vi "Drive Begin.vi"() -> ()   [LabVIEW 2016]
uses:
  <vilib>/Rock Robotics/WPI/Joystick/WPI_JoystickDeviceEnum.ctl
  <vilib>/Rock Robotics/SystemInterfaces/DIO/FPGA_DIOChannel.ctl
  <vilib>/Rock Robotics/WPI/Encoder/WPI_EncoderType.ctl
  <vilib>/Rock Robotics/SystemInterfaces/DIO/FPGA_DIOPWMChannel.ctl
  <vilib>/Rock Robotics/WPI/SafetyOutput/WPI_SafetyOutputConfigMenu.ctl
  <vilib>/Rock Robotics/WPI/Counter/WPI_CounterDigitalInputToDigitalSource.vi
  <vilib>/Rock Robotics/WPI/Utilities/WPI_GetSetVariantRefNum.vi
  <vilib>/Rock Robotics/WPI/RobotDrive/WPI_RobotDriveOpen2MotorWithVictorSP.vi
  <vilib>/Rock Robotics/WPI/Solenoid/WPI_SolenoidChannel.ctl
  <vilib>/Rock Robotics/WPI/Solenoid/WPI_SolenoidOpenSingle.vi
panel:
  out "error out":errorcluster
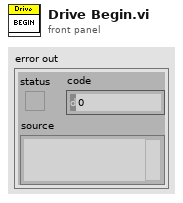
[diagram p1: front panel]
types:
  T1 = typedef "WPI_SafetyOutputConfigMenu.ctl" = enum16{"Enable", "Disable"}
  T2 = typedef "FPGA_DIOPWMChannel.ctl" = enum8{"PWM 0", "PWM 1", "PWM 2", "PWM 3", "PWM 4", "PWM 5", "PWM 6", "PWM 7", "PWM 8", "PWM 9", "PWM MXP 0", "PWM MXP 1", "PWM MXP 2", "PWM MXP 3", "PWM MXP 4", "PWM MXP 5", "PWM MXP 6", "PWM MXP 7", "PWM MXP 8", "PWM MXP 9", "Invalid"}
  T3 = typedef "FPGA_DIOChannel.ctl" = enum8{"DIO 0", "DIO 1", "DIO 2", "DIO 3", "DIO 4", "DIO 5", "DIO 6", "DIO 7", "DIO 8", "DIO 9", "DIO MXP 0", "DIO MXP 1", "DIO MXP 2", "DIO MXP 3", "DIO MXP 4", "DIO MXP 5", "DIO MXP 6", "DIO MXP 7", "DIO MXP 8", "DIO MXP 9", "DIO MXP 10", "DIO MXP 11", "DIO MXP 12", "DIO MXP 13", "DIO MXP 14", "DIO MXP 15", "SPI Port CS1", "SPI Port CS2", "SPI Port CS3", "SPI Port MISO", "SPI Port MOSI", "Invalid"}
  T4 = typedef "WPI_EncoderType.ctl" = enum16{"1x", "2x", "4x"}
  T5 = typedef "WPI_JoystickDeviceEnum.ctl" = enum16{"USB 0", "USB 1", "USB 2", "USB 3", "USB 4", "USB 5"}
  T6 = typedef "WPI_JoystickDevRef.ctl" = cluster{"Device":T5}
  T7 = typedef "WPI_SolenoidChannel.ctl" = enum8{"Solenoid 0", "Solenoid 1", "Solenoid 2", "Solenoid 3", "Solenoid 4", "Solenoid 5", "Solenoid 6", "Solenoid 7", "Invalid"}
  T8 = typedef "WPI_SolenoidDevRef.ctl" = cluster{"DevStatus":errorcluster, "Pneumatics Control Module":u8, "Forward Solenoid Channel":T7, "Reverse Solenoid Channel":T7}
  T9 = typedef "WPI_CompressorDevRef.ctl" = cluster{"DevStatus":errorcluster, "Pneumatics Control Module":u8}
  T10 = typedef "WPI_DigitalInputDevRef.ctl" = cluster{"DevStatus":errorcluster, "DIO Channel":T3}
  T11 = typedef "WPI_RobotDriveDevRef.ctl" = cluster{"DevStatus":errorcluster, "Motors[]":T12[], "Square Inputs":bool, "Max Output":dbl}
  T12 = typedef "WPI_MotorControlDeviceRef.ctl" = cluster{"DeviceStatus":errorcluster, "Type":T13, "PWM":cluster{"PWM Channel":T2, "DeadBand":T14}, "CAN":cluster{"Device Number":u8, "SetOutput VI Ref":variant, "GetOutput VI Ref":variant, "Enable VI Ref":variant, "Disable VI Ref":variant, "Data":variant}, "Invert":bool}
  T13 = typedef "WPI_MotorControlType.ctl" = enum16{"PWM", "CAN"}
  T14 = typedef "WPI_PWMDeadband.ctl" = cluster{"Name":string, "maxPositivePwm":i32, "minPositivePwm":i32, "centerPwm":i32, "maxNegativePwm":i32, "minNegativePwm":i32, "angularRange":u16}
  T15 = typedef "FPGA_CounterEncoderSourceConvertionLVSourceType.ctl" = cluster{"DevStatus":errorcluster, "AnalogTriggerMode?":bool, "DigitalMode":cluster{"DIO Channel":T16}, "AnalogTriggerMode":cluster{"AnalogTriggerIndex":T17, "OutputType":T18}}
  T16 = typedef "FPGA_DIODigitalSourceChannel.ctl" = enum8{"DIO 0", "DIO 1", "DIO 2", "DIO 3", "DIO 4", "DIO 5", "DIO 6", "DIO 7", "DIO 8", "DIO 9", "DIO MXP 0", "DIO MXP 1", "DIO MXP 2", "DIO MXP 3", "DIO MXP 4", "DIO MXP 5", "DIO MXP 6", "DIO MXP 7", "DIO MXP 8", "DIO MXP 9", "DIO MXP 10", "DIO MXP 11", "DIO MXP 12", "DIO MXP 13", "DIO MXP 14", "DIO MXP 15", "Disabled"}
  T17 = typedef "FPGA_AnalogTriggerIndex.ctl" = enum8{"Trig 0", "Trig 1", "Trig 2", "Trig 3", "Trig 4", "Trig 5", "Trig 6", "Trig 7", "Invalid"}
  T18 = typedef "FPGA_AnalogTriggerOutType.ctl" = enum16{"InWindow", "TriggerState", "Rising", "Falling"}
  T19 = typedef "WPI_EncoderDevRef.ctl" = cluster{"DevStatus":errorcluster, "EncoderIndex":T20, "CounterIndex":T21, "DistancePerCount":dbl, "Decoding Type":T4}
  T20 = typedef "FPGA_EncoderIdx.ctl" = enum8{"Enc 0", "Enc 1", "Enc 2", "Enc 3", "Enc 4", "Enc 5", "Enc 6", "Enc 7", "Invalid"}
  T21 = typedef "FPGA_CounterCtrSystemIndex.ctl" = enum8{"Ctr 0", "Ctr 1", "Ctr 2", "Ctr 3", "Ctr 4", "Ctr 5", "Ctr 6", "Ctr 7", "Invalid"}
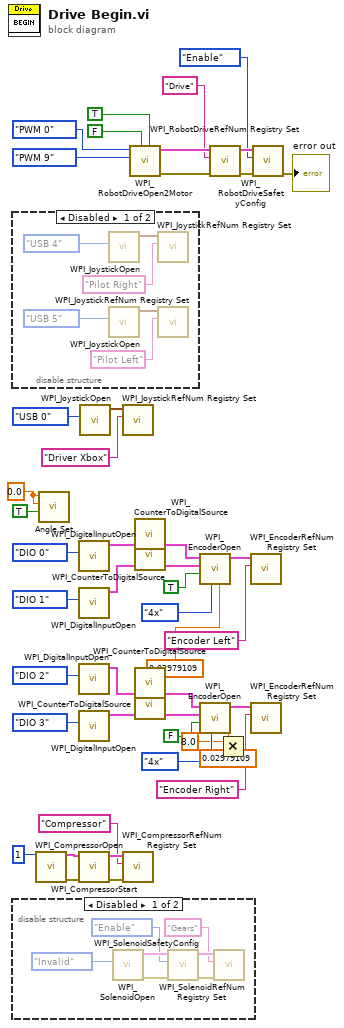
[diagram p0: block diagram]
diagram:
  w16 = 0.0 ("Angle Set")
  n1 = disable-structure shown="Disabled" {
    frame Disabled {
      n2 = call <vilib>:"WPI_JoystickOpen.vi"("JoystickDevice"=WPI_JoystickDeviceEnum."USB 4") -> ("JoystickDevRef"=w49:T6)  [unwired: 10 in]
      n3 = call <vilib>:"WPI_JoystickOpen.vi"("JoystickDevice"=WPI_JoystickDeviceEnum."USB 5") -> ("JoystickDevRef"=w52:T6)  [unwired: 10 in]
      n4 = call <vilib>:"WPI_JoystickRefNum Registry Set.vi"("refnum name"="Pilot Right", "JoystickDevRef"=w49) -> ()  [unwired: 8 in, 2 out]
      n5 = call <vilib>:"WPI_JoystickRefNum Registry Set.vi"("refnum name"="Pilot Left", "JoystickDevRef"=w52) -> ()  [unwired: 8 in, 2 out]
    }
    frame Enabled {
    }
  }
  n6 = disable-structure shown="Disabled" {
    frame Disabled {
      n7 = call-poly <vilib>:"WPI_SolenoidOpen.vi"("Solenoid Channel"=WPI_SolenoidChannel."Invalid" ("Forward Solenoid Channel")) -> ("error out"=w59:errorcluster, "SolenoidDevRef"=w58:T8)  [unwired: 9 in]
      n8 = call <vilib>:"WPI_SolenoidSafetyConfig.vi"("error in (no error)"=w59, "mode"=WPI_SafetyOutputConfigMenu."Enable", "SolenoidDevRef"=w58) -> ("error out"=w57:errorcluster, "SolenoidDevRef"=w56:T8)  [unwired: 7 in]
      n9 = call <vilib>:"WPI_SolenoidRefNum Registry Set.vi"("error in (no error)"=w57, "refnum name"="Gears", "SolenoidDevRef"=w56) -> ()  [unwired: 7 in, 2 out]
    }
    frame Enabled {
    }
  }
  n10 = call <vilib>:"WPI_CompressorOpen.vi"("Pneumatics Control Module (0)"=u8 1) -> ("CompressorDevRef"=w22:T9, "error out"=w23:errorcluster)  [unwired: 13 in]
  n11 = call "Angle Set.vi"("Set Angle?"=TRUE, "Angle Set"=w16, "Angle In"=w16) -> ()  [unwired: 8 in, 1 out]
  n12 = call <vilib>:"WPI_DigitalInputOpen.vi"("DIO Channel"=FPGA_DIOChannel."DIO 0" ("A Channel")) -> ("DigitalInputDevRef"=w30:T10)  [unwired: 2 in, 8 out]
  n13 = call <vilib>:"WPI_DigitalInputOpen.vi"("DIO Channel"=FPGA_DIOChannel."DIO 1" ("B Channel")) -> ("DigitalInputDevRef"=w29:T10)  [unwired: 2 in, 8 out]
  n14 = call <vilib>:"WPI_DigitalInputOpen.vi"("DIO Channel"=FPGA_DIOChannel."DIO 2" ("A Channel")) -> ("DigitalInputDevRef"=w41:T10)  [unwired: 2 in, 8 out]
  n15 = call <vilib>:"WPI_DigitalInputOpen.vi"("DIO Channel"=FPGA_DIOChannel."DIO 3" ("B Channel")) -> ("DigitalInputDevRef"=w42:T10)  [unwired: 2 in, 8 out]
  n16 = call <vilib>:"WPI_CompressorStart.vi"("error in (no error)"=w23, "CompressorDevRef"=w22) -> ("error out"=w20:errorcluster, "CompressorDevRef"=w21:T9)  [unwired: 8 in]
  n17 = call <vilib>:"WPI_JoystickOpen.vi"("JoystickDevice"=WPI_JoystickDeviceEnum."USB 0") -> ("JoystickDevRef"=w46:T6)  [unwired: 10 in]
  n18 = call <vilib>:"WPI_JoystickRefNum Registry Set.vi"("refnum name"="Driver Xbox", "JoystickDevRef"=w46) -> ()  [unwired: 8 in, 2 out]
  n19 = call <vilib>:"WPI_CompressorRefNum Registry Set.vi"("error in (no error)"=w20, "refnum name"="Compressor", "CompressorDevRef"=w21) -> ()  [unwired: 7 in, 2 out]
  n20 = call-poly <vilib>:"WPI_RobotDriveOpen2Motor.vi"("Right Motor Inverted"=TRUE ("Rear Right Motor Inverted"), "Left Motor Inverted"=FALSE ("Rear Left Motor Inverted"), "Right Motor"=FPGA_DIOPWMChannel."PWM 9" ("Rear Right Motor"), "Left Motor"=FPGA_DIOPWMChannel."PWM 0" ("Rear Left Motor")) -> ("error out"=w14:errorcluster, "RobotDriveDevRef"=w13:T11)  [unwired: 6 in]
  n21 = call-poly <vilib>:"WPI_CounterToDigitalSource.vi"("DigitalInputDevRef"=w30) -> ("Digital Source"=w31:T15)  [unwired: 6 out]
  n22 = call-poly <vilib>:"WPI_CounterToDigitalSource.vi"("DigitalInputDevRef"=w29) -> ("Digital Source"=w28:T15)  [unwired: 6 out]
  n23 = call-poly <vilib>:"WPI_CounterToDigitalSource.vi"("DigitalInputDevRef"=w41) -> ("Digital Source"=w40:T15)  [unwired: 6 out]
  n24 = call-poly <vilib>:"WPI_CounterToDigitalSource.vi"("DigitalInputDevRef"=w42) -> ("Digital Source"=w43:T15)  [unwired: 6 out]
  n25 = call <vilib>:"WPI_EncoderOpen.vi"("DistancePerCount"=0.02979109, "Decoding Type"=WPI_EncoderType."4x", "Invert Direction (False)"=TRUE ("Invert Direction"), "BSource"=w28, "ASource"=w31) -> ("EncoderDevRef"=w25:T19)  [unwired: 3 in, 3 out]
  n26 = call <vilib>:"WPI_RobotDriveRefNum Registry Set.vi"("error in (no error)"=w14, "refnum name"="Drive", "RobotDriveDevRef"=w13) -> ("error out"=w8:errorcluster, "RobotDriveDevRef"=w9:T11)  [unwired: 7 in]
  n27 = Multiply(x=8.0, y=0.02979109 ("DistancePerCount")) -> (x*y=w2:dbl)
  n28 = call <vilib>:"WPI_EncoderOpen.vi"("DistancePerCount"=w2, "Decoding Type"=WPI_EncoderType."4x", "Invert Direction (False)"=FALSE ("Invert Direction"), "BSource"=w43, "ASource"=w40) -> ("EncoderDevRef"=w27:T19)  [unwired: 3 in, 3 out]
  n29 = call <vilib>:"WPI_EncoderRefNum Registry Set.vi"("refnum name"="Encoder Left", "EncoderDevRef"=w25) -> ()  [unwired: 8 in, 2 out]
  n30 = call <vilib>:"WPI_EncoderRefNum Registry Set.vi"("refnum name"="Encoder Right", "EncoderDevRef"=w27) -> ()  [unwired: 8 in, 2 out]
  n31 = call <vilib>:"WPI_RobotDriveSafetyConfig.vi"("error in (no error)"=w8, "mode"=WPI_SafetyOutputConfigMenu."Enable", "RobotDriveDevRef"=w9) -> ("error out"=→"error out":errorcluster)  [unwired: 7 in, 1 out]
